vi "Names 2 Outputs.vi"(4 "Final  Output In":T1, 5 "Final  Output":T2) -> (2 "Final  Output Out":T1)   [LabVIEW 2013]
uses:
  Type Defs/Final Output for Dispaly 2.ctl
  Type Defs/Named Final Output name list with 02.ctl
panel:
  # "Channel A"
  # "Channel B"
  # "Channel C"
  # "Channel D"
  # "Channel A"
  # "Channel B"
  # "Channel C"
  # "Channel D"
  # "Channel A"
  # "Channel B"
  # "Channel C"
  # "Channel D"
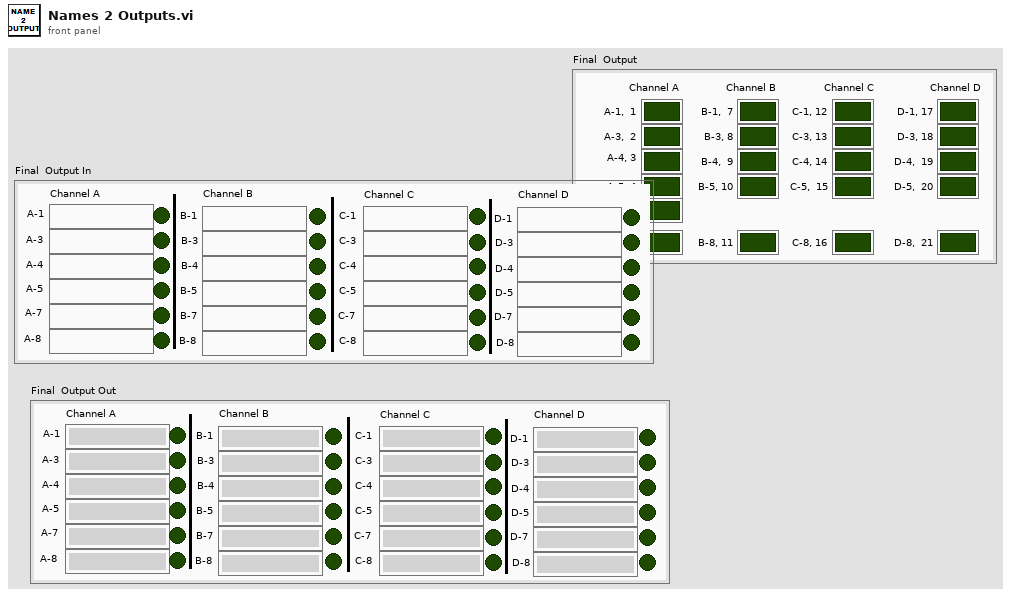
[diagram p1: front panel]
types:
  T1 = typedef "Named Final Output name list with 02.ctl" = cluster{"A-1,  1":string, "A-3,  2":string, "A-4, 3":string, "A-5, 4":string, "A-7, 5":string, "A-8, 6":string, "B-1,  7":string, "B-3, 8":string, "B-4,  9":string, "B-5, 10":string, "B-8, 11":string, "C-1, 12":string, "C-3, 13":string, "C-4, 14":string, "C-5,  15":string, "C-8, 16":string, "D-1, 17":string, "D-3, 18":string, "D-4,  19":string, "D-5,  20":string, "D-8,  21":string, "B-7":string, "C-7":string, "D-7":string, "A-1":bool, "A-3":bool, "A-4":bool, "A-5":bool, "A-7":bool, "A-8":bool, "B-1":bool, "B-3":bool, "B-4":bool, "B-5":bool, "B-7":bool, "B-8":bool, "C-1":bool, "C-3":bool, "C-4":bool, "C-5":bool, "C-7":bool, "C-8":bool, "D-1":bool, "D-3":bool, "D-4":bool, "D-5":bool, "D-7":bool, "D-8":bool}
  T2 = typedef "Final Output for Dispaly 2.ctl" = cluster{"A-1,  1":bool, "A-3,  2":bool, "A-4, 3":bool, "A-5, 4":bool, "ABCD-7, 5":bool, "A-8, 6":bool, "B-1,  7":bool, "B-3, 8":bool, "B-4,  9":bool, "B-5, 10":bool, "B-8, 11":bool, "C-1, 12":bool, "C-3, 13":bool, "C-4, 14":bool, "C-5,  15":bool, "C-8, 16":bool, "D-1, 17":bool, "D-3, 18":bool, "D-4,  19":bool, "D-5,  20":bool, "D-8,  21":bool}
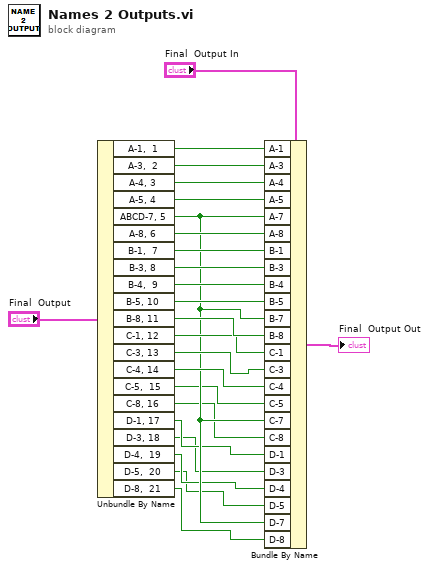
[diagram p0: block diagram]
diagram:
  n1 = Unbundle By Name("Final  Output") -> ("A-1,  1"=w22:bool, "A-3,  2"=w21:bool, "A-4, 3"=w20:bool, "A-5, 4"=w19:bool, "ABCD-7, 5"=w8:bool, "A-8, 6"=w18:bool, "B-1,  7"=w17:bool, "B-3, 8"=w16:bool, "B-4,  9"=w15:bool, "B-5, 10"=w13:bool, "B-8, 11"=w12:bool, "C-1, 12"=w11:bool, "C-3, 13"=w10:bool, "C-4, 14"=w9:bool, "C-5,  15"=w7:bool, "C-8, 16"=w6:bool, "D-1, 17"=w5:bool, "D-3, 18"=w4:bool, "D-4,  19"=w3:bool, "D-5,  20"=w2:bool, "D-8,  21"=w1:bool)
  n2 = Bundle By Name(cluster="Final  Output In", "A-1"=w22, "A-3"=w21, "A-4"=w20, "A-5"=w19, "A-7"=w8, "A-8"=w18, "B-1"=w17, "B-3"=w16, "B-4"=w15, "B-5"=w13, "B-7"=w8, "B-8"=w12, "C-1"=w11, "C-3"=w10, "C-4"=w9, "C-5"=w7, "C-7"=w8, "C-8"=w6, "D-1"=w5, "D-3"=w4, "D-4"=w3, "D-5"=w2, "D-7"=w8, "D-8"=w1) -> (→"Final  Output Out":T1)
